vi "DigitizerConfig.vi"(5 "ExportTrigger? (F)":bool, 7 "Config Trigger? (T)":bool=TRUE, 8 "error in (no error)":errorcluster, 10 "FLImDAQ":T1={"Digitizer 1"="PXI1Slot3", "Digitizer 2"="PXI1Slot4", "Channel"=enum."Channel 0", "trigger source"="VAL_EXTERNAL", "trigger level"=0.5, "trigger delay"=1.35e-07, "min sample rate"=12500000000.0, "min record length"=2500, "vertical range"=1.0, "vertical offset"=-0.25, "Waveform to Avg"=2000} caption="FLIm DAQ Configuration" {"trigger delay" format="%^#.4e"; "trigger level" min=0.0 max=3.5 step=0.5 format="%.2f"; "vertical offset" format="%.4f"; "vertical range" format="%.2f"; "min sample rate" format="%#.2p"}, 11 "IVI Refnum in":refnum<k15>) -> (0 "error out":errorcluster, 3 "IVI Refnum out":refnum<k15>)   [LabVIEW 2024]
uses:
  FLImDAQ.ctl
  <instrlib>/niScope/Controls/niScope trigger source.ctl
  <instrlib>/niScope/Controls/niScope vertical coupling.ctl
  <instrlib>/niScope/Controls/niScope acquisition type.ctl
  <instrlib>/niScope/Controls/niScope trigger coupling.ctl
  <instrlib>/niScope/Controls/niScope trigger slope.ctl
  <instrlib>/niScope/Controls/niScope exportable signals.ctl
  <instrlib>/niScope/Controls/niScope export destinations.ctl
  <instrlib>/niScope/Configure/Trigger/niScope Configure Trigger Edge.vi
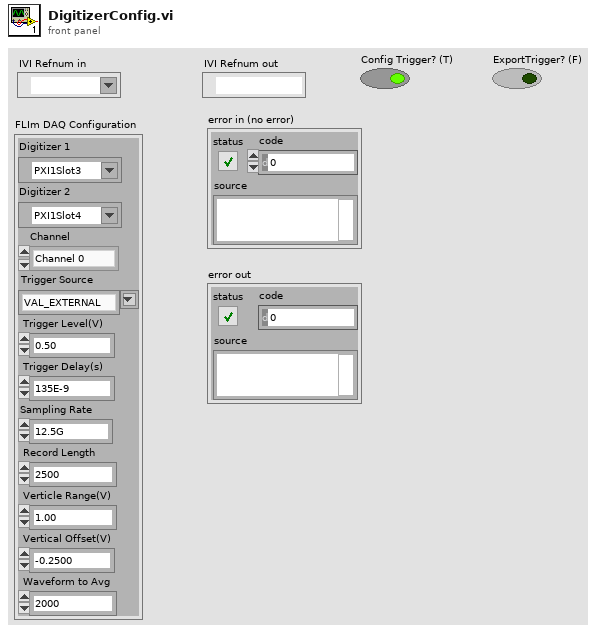
[diagram p1: front panel]
types:
  T1 = typedef "FLImDAQ.ctl" = cluster{"Digitizer 1":refnum<k15>, "Digitizer 2":refnum<k15>, "Channel":enum16{"Channel 0", "Channel 1", "Channel 0&1"}, "trigger source":T2, "trigger level":dbl, "trigger delay":dbl, "min sample rate":dbl, "min record length":i32, "vertical range":dbl, "vertical offset":dbl, "Waveform to Avg":i16}
  T2 = typedef "niScope trigger source.ctl" = string
  T3 = typedef "niScope export destinations.ctl" = string
  T4 = typedef "niScope acquisition type.ctl" = i32
  T5 = typedef "niScope vertical coupling.ctl" = i32
  T6 = typedef "niScope trigger slope.ctl" = i32
  T7 = typedef "niScope trigger coupling.ctl" = u16
  T8 = typedef "niScope exportable signals.ctl" = u16
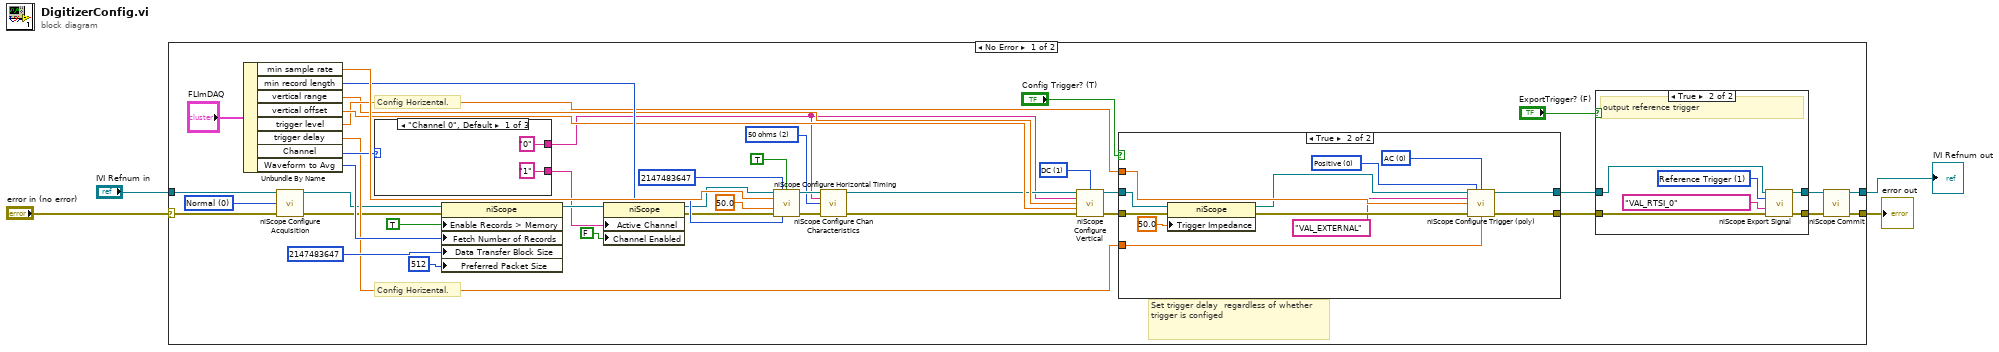
[diagram p0: block diagram]
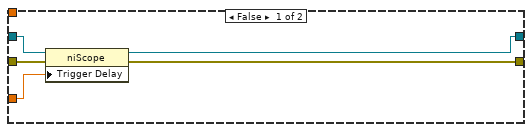
[diagram p3: hidden frame]
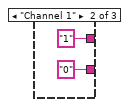
[diagram p4: hidden frame]
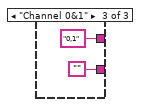
[diagram p5: hidden frame]
diagram:
  n1 = case shown="No Error" "error in (no error)" {
    selector: "error in (no error)" -> [w11 w79]
    tunnel: [w46 w78] -> w4
    tunnel: [w39 w79] -> w3
    tunnel: "IVI Refnum in" -> [w13 w78]
    frame No Error {
      w14 = T4 0 items=["Normal"=0, "Flex Res"=1, "DDC"=3] ("acquisition Type")
      w31 = u32 2 items=["1 mega ohm"=0, "50 ohms"=2] ("input impedance")
      w43 = T5 1 items=["AC", "DC", "Ground"] ("vertical coupling")
      # "Set trigger delay  regardless of whether trigger is configed"
      # "Config Horizental."
      # "Config Horizental."
      n2 = Unbundle By Name("FLImDAQ") -> ("min sample rate"=w45:dbl, "min record length"=w44:i32, "vertical range"=w40:dbl, "vertical offset"=w42:dbl, "trigger level"=w41:dbl, "trigger delay"=w15:dbl, "Channel"=w37:enum16{"Channel 0", "Channel 1", "Channel 0&1"}, "Waveform to Avg"=w24:i16)
      n3 = call <instrlib>:"niScope Configure Acquisition.vi"("instrument handle"=w13, "acquisition Type"=w14, "error in"=w11) -> ("instrument handle out"=w12:refnum<k15>, "error out"=w10:errorcluster)  [unwired: 11 in]
      n4 = case shown="\"Channel 0\", Default" w37 {
        tunnel: ["0" ("channels") "1" ("channels") "0,1" ("channels")] -> w23
        tunnel: ["1" ("channels") "0" ("channels") ""] -> w21
        frame "Channel 0", Default {
        }
        frame "Channel 1" {
        }
        frame "Channel 0&1" {
        }
      }
      n5 = property class="niScope"(reference=w12, error in=w10, "Enable Records > Memory"=TRUE ("Horizontal:Enable Records > Memory"), "Fetch Number of Records"=w24, "Data Transfer Block Size"=2147483647 ("Fetch:Data Transfer Block Size"), "Preferred Packet Size"=512 ("Fetch:Advanced:Preferred Packet Size")) -> (reference out=w22:refnum<k15>)  [unwired: 1 out]
      n6 = property class="niScope"(reference=w22, "Active Channel"=w21, "Channel Enabled"=FALSE ("Vertical:Channel Enabled")) -> (reference out=w19:refnum<k15>, error out=w18:errorcluster)  [unwired: 1 in]
      n7 = call <instrlib>:"niScope Configure Horizontal Timing.vi"("instrument handle"=w19, "number of records"=2147483647, "enforce realtime"=TRUE, "min sample rate"=w45, "reference position"=50.0, "error in"=w18, "min record length"=w44) -> ("instrument handle out"=w35:refnum<k15>, "error out"=w33:errorcluster)  [unwired: 7 in]
      n8 = call <instrlib>:"niScope Configure Chan Characteristics.vi"("instrument handle"=w35, "channels"=w23, "input impedance"=w31, "error in"=w33) -> ("instrument handle out"=w34:refnum<k15>, "error out"=w32:errorcluster)  [unwired: 10 in]
      n9 = call <instrlib>:"niScope Configure Vertical.vi"("instrument handle"=w34, "vertical coupling"=w43, "channels"=w23, "vertical range"=w40, "vertical offset"=w42, "error in"=w32) -> ("instrument handle out"=w17:refnum<k15>, "error out"=w16:errorcluster)  [unwired: 8 in]
      n10 = case shown="True" "Config Trigger? (T)" {
        tunnel: w17 -> [w59 w67]
        tunnel: w41 -> [_ w71]
        tunnel: w16 -> [w56 w65]
        tunnel: [w58 w63] -> w9
        tunnel: [w55 w62] -> w7
        tunnel: w15 -> [w57 w69]
        frame False {
          n11 = property class="niScope"(reference=w59, error in=w56, "Trigger Delay"=w57) -> (reference out=w58:refnum<k15>, error out=w55:errorcluster)
        }
        frame True {
          w68 = T6 0 items=["Positive", "Negative"] ("trigger slope")
          w70 = T7 0 items=["AC"=0, "DC"=1, "HF Reject"=3, "LF Reject"=4, "AC Plus HF Reject"=1001] ("trigger coupling")
          n12 = property class="niScope"(reference=w67, error in=w65, "Trigger Impedance"=50.0 ("Triggering:Trigger Impedance")) -> (reference out=w66:refnum<k15>, error out=w64:errorcluster)
          n13 = call-poly <instrlib>:"niScope Configure Trigger (poly).vi"("instrument handle"=w66, "trigger slope"=w68, "trigger coupling"=w70, "trigger source"=T2 "VAL_EXTERNAL", "trigger level"=w71, "error in"=w64, "trigger delay"=w69) -> ("instrument handle out"=w63:refnum<k15>, "error out"=w62:errorcluster)  [unwired: 7 in]
        }
      }
      n14 = case shown="True" "ExportTrigger? (F)" {
        tunnel: w9 -> [w48 w54]
        tunnel: [w48 w53] -> w8
        tunnel: w7 -> [w47 w52]
        tunnel: [w47 w51] -> w6
        frame False {
        }
        frame True {
          w50 = T8 1 items=["None"=0, "Start Trigger"=2, "Advance Trigger"=5, "Reference Trigger"=1, "End of Record Event"=4, "End of Acquisition Event"=3, "Ready for Start Event"=7, "Ready for Advance Event"=6, "Ready for Reference Event"=10, "Reference Clock"=100, "Sample Clock"=101, "5 Volt Power"=13] ("signal")
          # "output reference trigger"
          n15 = call <instrlib>:"niScope Export Signal.vi"("instrument handle"=w54, "signal"=w50, "output terminal"=T3 "VAL_RTSI_0", "error in"=w52) -> ("instrument handle out"=w53:refnum<k15>, "error out"=w51:errorcluster)  [unwired: 10 in]
        }
      }
      n16 = call <instrlib>:"niScope Commit.vi"("instrument handle"=w8, "error in"=w6) -> ("instrument handle out"=w46:refnum<k15>, "error out"=w39:errorcluster)  [unwired: 12 in]
    }
    frame Error {
    }
  }
  "IVI Refnum out" <- w4
  "error out" <- w3
